vi "Slew Rate.vi"(8 "错误输入（无错误）":errorcluster, 11 "Analog Waveforms":waveform(dbl)[](array[waveform])) -> (0 "错误输出":errorcluster, 2 "Dynamic Data":dynamicdata(waveform), 3 "waveform":waveform(dbl))   [LabVIEW 2019]
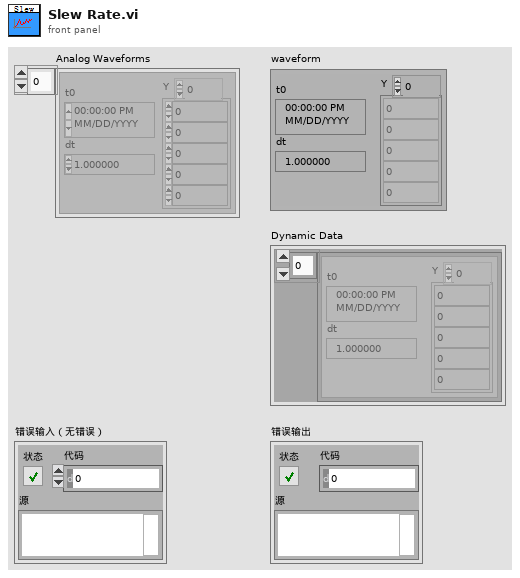
[diagram p1: front panel]
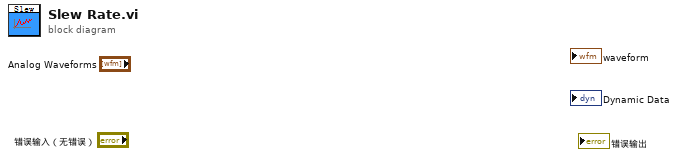
[diagram p0: block diagram]
diagram:
